vi "source_final_beep.vi"(8 "error in (no error)":errorcluster, 11 "VISA resource name":refnum<visa-resource-name>) -> (0 "error out":errorcluster, 3 "VISA resource name out":refnum<visa-resource-name>)   [LabVIEW 2020]
doc: "Plays a tone when the measurement is finished."
uses:
  <instrlib>/Keithley 24XX/Keithley 24XX.lvlib
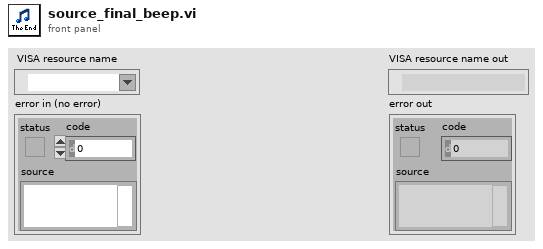
[diagram p1: front panel]
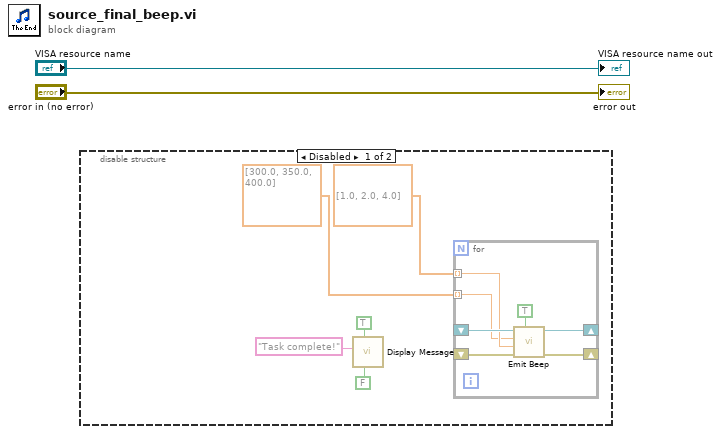
[diagram p0: block diagram]
diagram:
  n1 = disable-structure shown="Disabled" {
    frame Disabled {
      n2 = call <instrlib>:"Display Message.vi"("Enable Lower Message (T: Enable)"=FALSE, "Enable Upper Message (T: Enable)"=TRUE, "Upper Message (\"Default\")"="Task complete!" ("Upper Message (\"Default\")")) -> ()  [unwired: 7 in, 2 out]
      n3 = for {
        shift-right: [w12] -> _
        shift-left: _ -> [w14]
        shift-right: [w11] -> _
        shift-left: _ -> [w13]
        tunnel: dbl[] [300.0, 350.0, 400.0] -> [w9] mode=indexing
        tunnel: dbl[] [1.0, 2.0, 4.0] -> [w10] mode=indexing
        n4 = call <instrlib>:"Emit Beep.vi"("Enable Beep (F)"=TRUE, "error in (no error)"=w13, "Beep Duration (.25 s)"=w10, "Beep Frequency (300)"=w9, "VISA resource name"=w14) -> ("error out"=w11:errorcluster, "VISA resource name out"=w12:refnum<visa-resource-name>)  [unwired: 5 in]
      }
    }
    frame Enabled {
    }
  }
  "VISA resource name out" <- "VISA resource name"
  "error out" <- "error in (no error)"
